vi "Example - Multiple Loggers.vi"() -> ()   [LabVIEW 2016, in "Global_logger.lvlib"]
doc: "Example of logging into UI elements."
uses:
  Global_logger.lvlib
  UI Options.ctl
  General Options.ctl
  Log Fields.ctl
  Level Meaning.ctl
  Sorting.ctl
  New UI Logger.vi
panel:
  in  "Table Control":string[][](table)
  in  "Multicolumn Listbox":i32(listbox)=-1
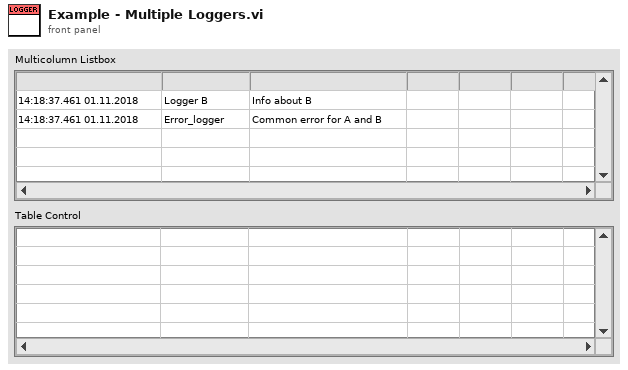
[diagram p1: front panel]
types:
  T1 = typedef "Global_logger.lvlib/General Options.ctl" = cluster{"Format":T2[], "Timestamp format":string, "Level Meaning":T3, "Sorting":T4}
  T2 = typedef "Global_logger.lvlib/Log Fields.ctl" = enum16{"Timestamp", "Level", "Message", "Source VI", "Source App", "Logger Name"}
  T3 = typedef "Global_logger.lvlib/Level Meaning.ctl" = enum16{"Standard", "Positive", "Exact"}
  T4 = typedef "Global_logger.lvlib/Sorting.ctl" = enum16{"Add to Bottom", "Add to Top"}
  T5 = typedef "Global_logger.lvlib/UI Options.ctl" = cluster{"Ctl Refnum":refnum<vi>, "Delimiter":string}
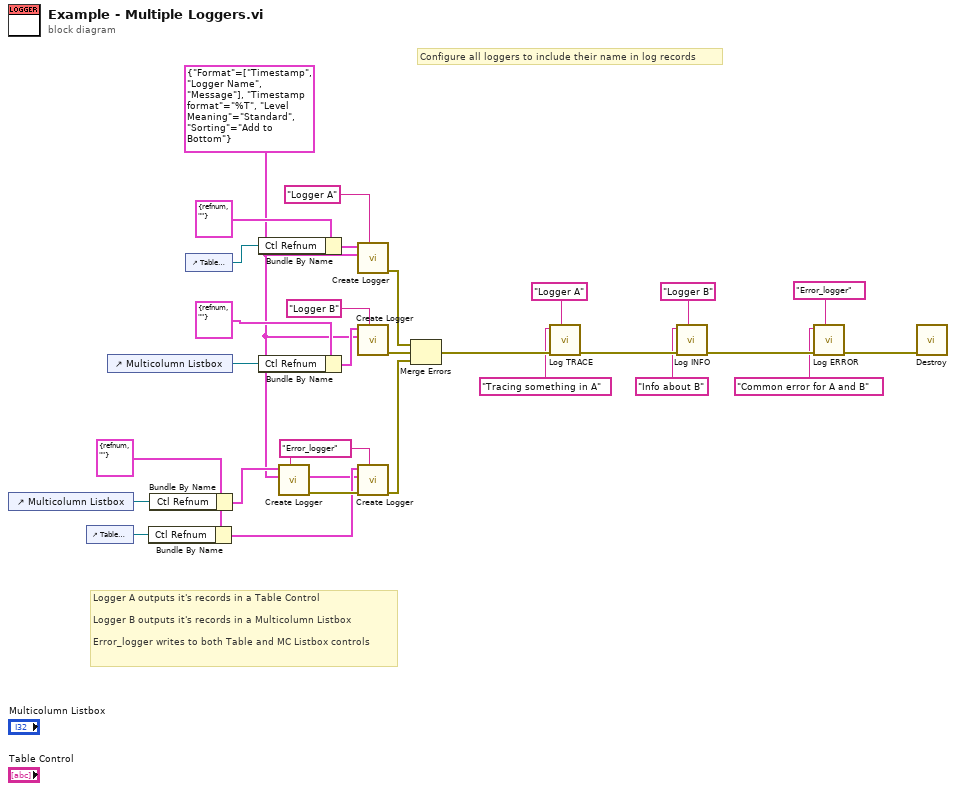
[diagram p0: block diagram]
diagram:
  w3 = T1 {"Format"=[enum."Timestamp", enum."Logger Name", enum."Message"], "Timestamp format"="%T", "Level Meaning"=enum."Standard", "Sorting"=enum."Add to Bottom"} ("General Options")
  w11 = "Error_logger" ("Logger Name")
  w10 = T5 {"Ctl Refnum"=refnum, "Delimiter"=""} ("UI Options")
  # "Logger A outputs it's records in a Table Control\n\nLogger B outputs it's records in a Multicolumn Listbox\n\nError_logger writes to both Table and MC Listbox controls"
  # "Configure all loggers to include their name in log records"
  n1 = control-ref of="Multicolumn Listbox"() -> (w14:refnum<vi>)
  n2 = control-ref of="Table Control"() -> (w8:refnum<vi>)
  n3 = control-ref of="Multicolumn Listbox"() -> (w29:refnum<vi>)
  n4 = Bundle By Name(cluster=w10, "Ctl Refnum"=w8) -> (w9:T5)
  n5 = Bundle By Name(cluster=w10, "Ctl Refnum"=w14) -> (w15:T5)
  n6 = control-ref of="Table Control"() -> (w27:refnum<vi>)
  n7 = Bundle By Name(cluster=T5 {"Ctl Refnum"=refnum, "Delimiter"=""} ("UI Options"), "Ctl Refnum"=w27) -> (w26:T5)
  n8 = Bundle By Name(cluster=T5 {"Ctl Refnum"=refnum, "Delimiter"=""} ("UI Options"), "Ctl Refnum"=w29) -> (w28:T5)
  n9 = call-poly "Create Logger.vi"("Logger Name"=w11, "General Options"=w3, "UI Options"=w15) -> ("error out"=w13:errorcluster)  [unwired: 8 in]
  n10 = call-poly "Create Logger.vi"("Logger Name"="Logger A", "General Options"=w3, "UI Options"=w26) -> ("error out"=w23:errorcluster)  [unwired: 8 in]
  n11 = call-poly "Create Logger.vi"("Logger Name"="Logger B", "General Options"=w3, "UI Options"=w28) -> ("error out"=w22:errorcluster)  [unwired: 8 in]
  n12 = call-poly "Create Logger.vi"("Logger Name"=w11, "error in (no error)"=w13, "General Options"=w3, "UI Options"=w9) -> ("error out"=w12:errorcluster)  [unwired: 7 in]
  n13 = Merge Errors(w23, w22, w12) -> (w19:errorcluster)
  n14 = call "Log TRACE.vi"("Logger Name"="Logger A", "error in (no error)"=w19, "Message"="Tracing something in A") -> ("error out"=w17:errorcluster)  [unwired: 8 in]
  n15 = call "Log INFO.vi"("Logger Name"="Logger B", "error in (no error)"=w17, "Message"="Info about B") -> ("error out"=w7:errorcluster)  [unwired: 8 in]
  n16 = call "Log ERROR.vi"("Logger Name"="Error_logger", "error in (no error)"=w7, "Message"="Common error for A and B") -> ("error out"=w6:errorcluster)  [unwired: 8 in]
  n17 = call "Destroy.vi"("error in (no error)"=w6) -> ()  [unwired: 10 in, 1 out]
